vi "Query Device ID.vi"(0 "3446X in":refnum<class "3446X.lvclass">, 11 "error in (no error)":errorcluster) -> (4 "3446X out":refnum<class "3446X.lvclass">, 6 "Model":string, 8 "Serial Number":string, 10 "Firmware":string, 15 "error out":errorcluster)   [LabVIEW 2018, in "3446X.lvlib" / "3446X.lvclass"]
uses:
  3446X.lvclass
  3446X.lvclass/3446X.ctl
  <instrlib>/Agilent 3446X Series/Agilent 3446X Series.lvlib
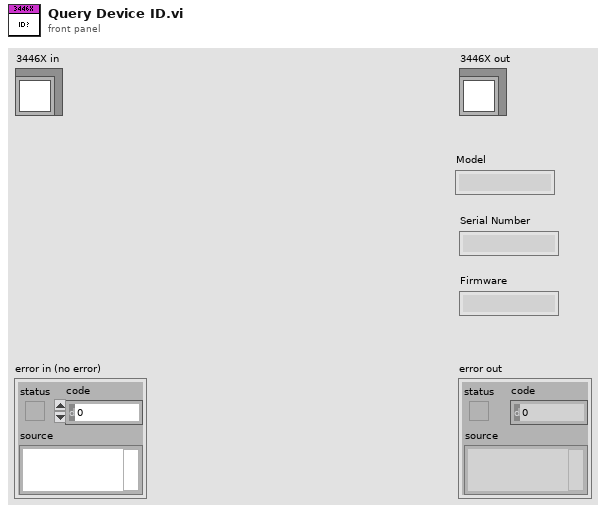
[diagram p1: front panel]
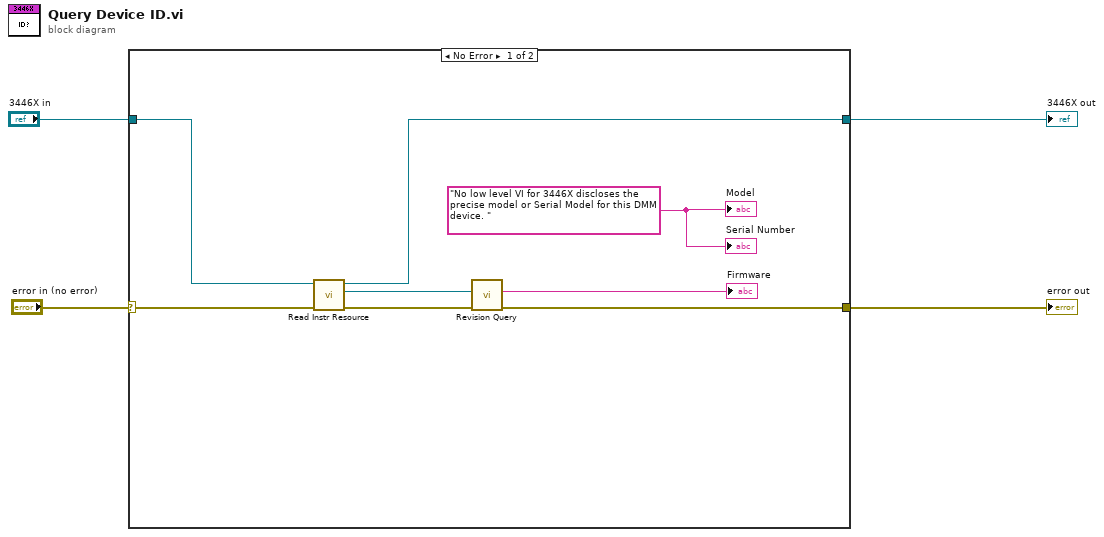
[diagram p0: block diagram]
diagram:
  n1 = case shown="No Error" "error in (no error)" {
    selector: "error in (no error)" -> [w12 w13]
    tunnel: [w10 w14] -> w3
    tunnel: "3446X in" -> [w11 w14]
    tunnel: [w6 w13] -> w1
    frame No Error {
      w5 = "No low level VI for 3446X discloses the precise model or Serial Model for this DMM device. "
      n2 = call "Read Instr Resource.vi"("error in (no error)"=w12, "3446X in"=w11) -> ("error out"=w8:errorcluster, "Instr Resource"=w9:refnum<visa-resource-name>, "3446X out"=w10:refnum<class "3446X.lvclass">)  [unwired: 7 in]
      n3 = call <instrlib>:"Revision Query.vi"("error in (no error)"=w8, "VISA resource name"=w9) -> ("error out"=w6:errorcluster, "Instrument Firmware Revision"=→"Firmware":string)  [unwired: 6 in, 2 out]
      "Model" <- w5
      "Serial Number" <- w5
    }
    frame Error {
    }
  }
  "error out" <- w1
  "3446X out" <- w3
